vi "CS++DMM-Readout.vi"() -> ()   [LabVIEW 2015, in "CS++DMM.lvlib"]
uses:
  CS++DMM.lvlib
  CSPP_Core/Classes/CS++BaseClasses/Factory/CS++Factory.lvclass
  CSPP_Core/Classes/CS++BaseClasses/Factory/CS++Factory.lvclass/CS++Factory.ctl
  CS++DMM.lvclass
  CSPP_Core/Actors/CS++DeviceActor/CS++DeviceActor.lvclass/CS++DeviceActor.ctl
  CSPP_Core/Actors/CS++DeviceActor/Read Resource Name.vi
  CSPP_Core/Actors/CS++DeviceActor/CS++DeviceActor.lvclass
panel:
  in  "CS++Object Names":string[](array[string])=["DMM3458A-GPIB0-21", "DMM3458A-GPIB0-22"]
  out "Last Time":timestamp format="%<%H:%M:%S%1u>T"
  in  "File Path Control":path=path "C:/User/Brand/LVP/STF/STF.ini"
  out "error out":errorcluster
  in  "Stop Button":bool
  out "Readings":dbl[](array[numeric])
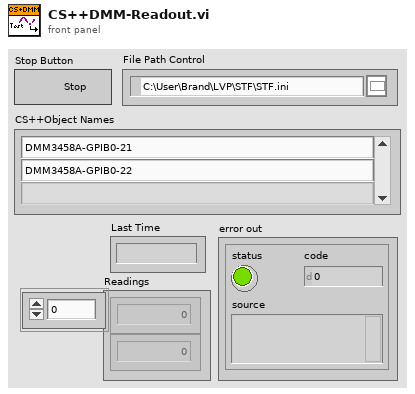
[diagram p1: front panel]
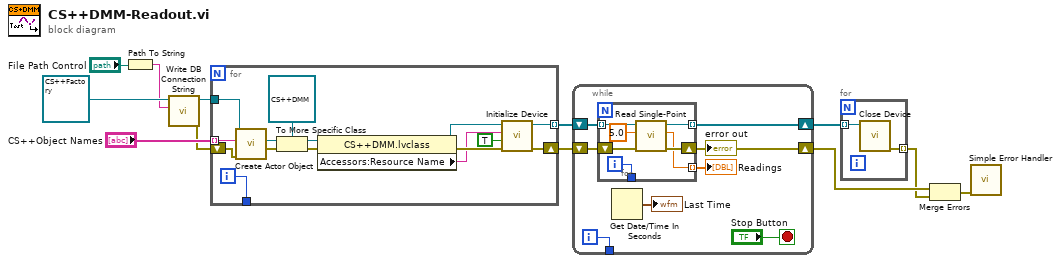
[diagram p0: block diagram]
diagram:
  n1 = Path To String(path="File Path Control") -> (string=w6:string)
  n2 = call "Write DB Connection String.vi"("DB Connection String"=w6, "CS++Factory in"=refnum<class "CS++Factory.lvclass"> refnum ("CS++BaseClasses.lvlib:CS++Factory.lvclass")) -> ("error out"=w1:errorcluster, "CS++Factory out"=w8:refnum<class "CS++Factory.lvclass">)  [unwired: 8 in]
  n3 = for {
    tunnel: w8 -> [w27]
    tunnel: "CS++Object Names" -> [w22] mode=indexing
    tunnel: [w13] -> w12 mode=indexing
    shift-right: [w14] -> w11
    shift-left: w1 -> [w16]
    tunnel: [w15] -> _
    i -> [w15]
    n4 = call "Create Actor Object.vi"("error in (no error)"=w16, "Object Name"=w22, "CS++Factory in"=w27) -> ("error out"=w25:errorcluster, "CS++BaseActor"=w26:refnum<class "CS++BaseActor.lvclass">)  [unwired: 5 in, 2 out]
    n5 = To More Specific Class(target class=refnum<class "CS++DMM.lvclass"> refnum ("CS++DMM.lvlib:CS++DMM.lvclass"), reference=w26, error in=w25) -> (specific class reference=w23:refnum<class "CS++DMM.lvclass">, error out=w20:errorcluster)
    n6 = property class="CS++DMM.lvclass"(reference=w23, error in=w20) -> (reference out=w21:refnum<class "CS++DMM.lvclass">, error out=w19:errorcluster, "Accessors:Resource Name"=w18:string)
    n7 = call "Initialize Device.vi"("error in (no error)"=w19, "Reset (F)"=TRUE, "Resource Name"=w18, "CS++DeviceActor in"=w21) -> ("error out"=w14:errorcluster, "CS++DeviceActor out"=w13:refnum<class "CS++DMM.lvclass">)  [unwired: 6 in]
  }
  n8 = while {
    shift-right: [w33] -> w5
    shift-left: w11 -> [w34]
    shift-right: [w32] -> w10
    shift-left: w12 -> [w35]
    tunnel: [w28] -> _
    i -> [w28]
    stop <- "Stop Button" stop-if-true
    n9 = for {
      tunnel: w35 -> [w42] mode=indexing
      tunnel: [w39] -> w32 mode=indexing
      shift-right: [w40] -> w33
      shift-left: w34 -> [w41]
      tunnel: [w38] -> w31 mode=indexing
      tunnel: [w36] -> _
      i -> [w36]
      n10 = call "Read Single-Point.vi"("error in (no error)"=w41, "maximum time (5s)"=dbl[unit] 5.0, "CS++DMM in"=w42) -> ("error out"=w40:errorcluster, "reading"=w38:dbl, "CS++DMM out"=w39:refnum<class "CS++DMM.lvclass">)  [unwired: 6 in]
    }
    "Readings" <- w31
    "error out" <- w33
    n11 = Get Date/Time In Seconds() -> (seconds since 1Jan1904=→"Last Time":timestamp)
  }
  n12 = for {
    tunnel: w10 -> [w44] mode=indexing
    tunnel: [w43] -> w4 mode=indexing
    n13 = call "Close Device.vi"("CS++DeviceActor in"=w44) -> ("error out"=w43:errorcluster)  [unwired: 9 in, 1 out]
  }
  n14 = Merge Errors(w5, w4) -> (w3:errorcluster)
  n15 = call <vilib>:"Simple Error Handler.vi"("error in (no error)"=w3) -> ()  [unwired: 4 in, 5 out]
